vi "Close-characteristics-files.vi"(8 "error in":errorcluster, 11 "Storage params. ref. in":refnum<data-value>) -> (0 "error IO":errorcluster, 1 "Succes?":bool, 3 "Storage params. ref.":refnum<data-value>)   [LabVIEW 2013, in "CameraVision.lvlib" / "CV-Storage.lvclass"]
doc: "This function closes the access references to the characteristics data file. This prevents further changes and allows the memory to be released.\n\nIn case the acquisition was aborted in the initialization phase, the references could be invalid. Invalid references are detected and ignored."
uses:
  CV-Storage.lvclass
  CV-Storage.lvclass/CV-Storage.ctl
  Read Characteristics file reference RW.vi
  Read Characteristics file reference RO.vi
  Read Temperature file reference W.vi
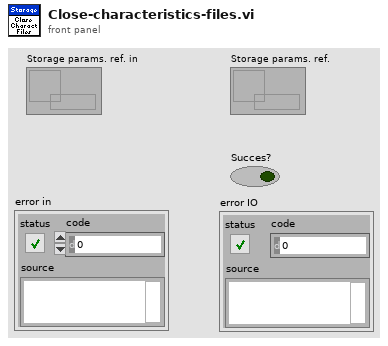
[diagram p1: front panel]
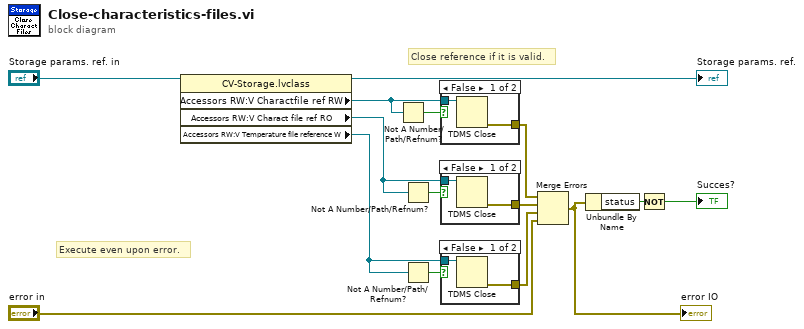
[diagram p0: block diagram]
diagram:
  # "Execute even upon error."
  # "Close reference if it is valid."
  n1 = property class="CV-Storage.lvclass"(reference="Storage params. ref. in") -> (reference out=→"Storage params. ref.":refnum<data-value>, "Accessors RW:V Charactfile ref RW"=w11:refnum<k34>, "Accessors RW:V Charact file ref RO"=w10:refnum<k34>, "Accessors RW:V Temperature file reference W"=w4:refnum<k34>)  [unwired: 1 in, 1 out]
  n2 = Not A Number/Path/Refnum?(number/path/refnum=w11) -> (NaN/Path/Refnum?=w7:bool)
  n3 = Not A Number/Path/Refnum?(number/path/refnum=w10) -> (NaN/Path/Refnum?=w6:bool)
  n4 = Not A Number/Path/Refnum?(number/path/refnum=w4) -> (NaN/Path/Refnum?=w5:bool)
  n5 = case shown="False" w7 {
    tunnel: [w17 _] -> w8
    tunnel: w11 -> [w16 _]
    frame False {
      n6 = TDMS Close(11:w16) -> (0:w17:errorcluster)  [unwired: 1 in, 1 out]
    }
    frame True {
    }
  }
  n7 = case shown="False" w6 {
    tunnel: w10 -> [w19 _]
    tunnel: [w18 _] -> w9
    frame False {
      n8 = TDMS Close(11:w19) -> (0:w18:errorcluster)  [unwired: 1 in, 1 out]
    }
    frame True {
    }
  }
  n9 = case shown="False" w5 {
    tunnel: w4 -> [w21 _]
    tunnel: [w20 _] -> w3
    frame False {
      n10 = TDMS Close(11:w21) -> (0:w20:errorcluster)  [unwired: 1 in, 1 out]
    }
    frame True {
    }
  }
  n11 = Merge Errors(w8, w9, w3, "error in") -> (w1:errorcluster)
  "error IO" <- w1
  n12 = Unbundle By Name(w1) -> ("status"=w12:bool)
  n13 = Not(x=w12) -> (.not. x?=→"Succes?":bool)
